vi "ADO Connection Set Mode.vi"(8 "error in (no error)":errorcluster, 10 "Mode":i32(ring) items=["adModeUnknown"=0, "adModeRead"=1, "adModeWrite"=2, "adModeReadWrite"=3, "adModeShareDenyRead"=4, "adModeShareDenyWrite"=8, "adModeShareExclusive"=12, "adModeShareDenyNone"=16, "adModeRecursive"=4194304], 11 "ADODB._Connection In":refnum<k7>) -> (0 "error out":errorcluster, 3 "ADODB._Connection Out":refnum<k7>)   [LabVIEW 2013]
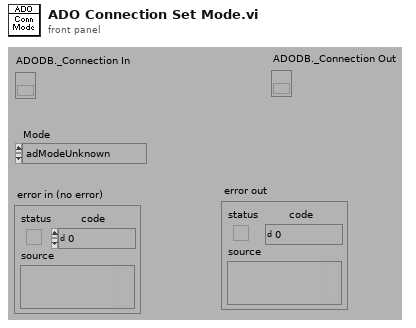
[diagram p1: front panel]
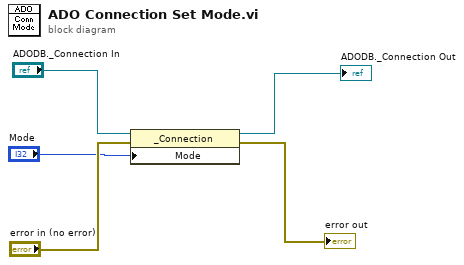
[diagram p0: block diagram]
diagram:
  n1 = property class="_Connection"(reference="ADODB._Connection In", error in="error in (no error)", "Mode"="Mode") -> (reference out=→"ADODB._Connection Out":refnum<k7>, error out=→"error out":errorcluster)
